vi "Indexed String To Enum.vi"(7 "Variant":variant, 8 "error in (no error)":errorcluster, 11 "String":string) -> (0 "error out":errorcluster, 3 "Enum":variant)   [LabVIEW 2017, in "ClusterCfgTable.lvlib"]
uses:
  ClusterCfgTable.lvlib
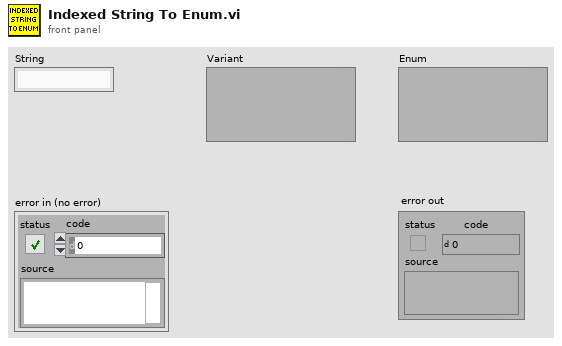
[diagram p1: front panel]
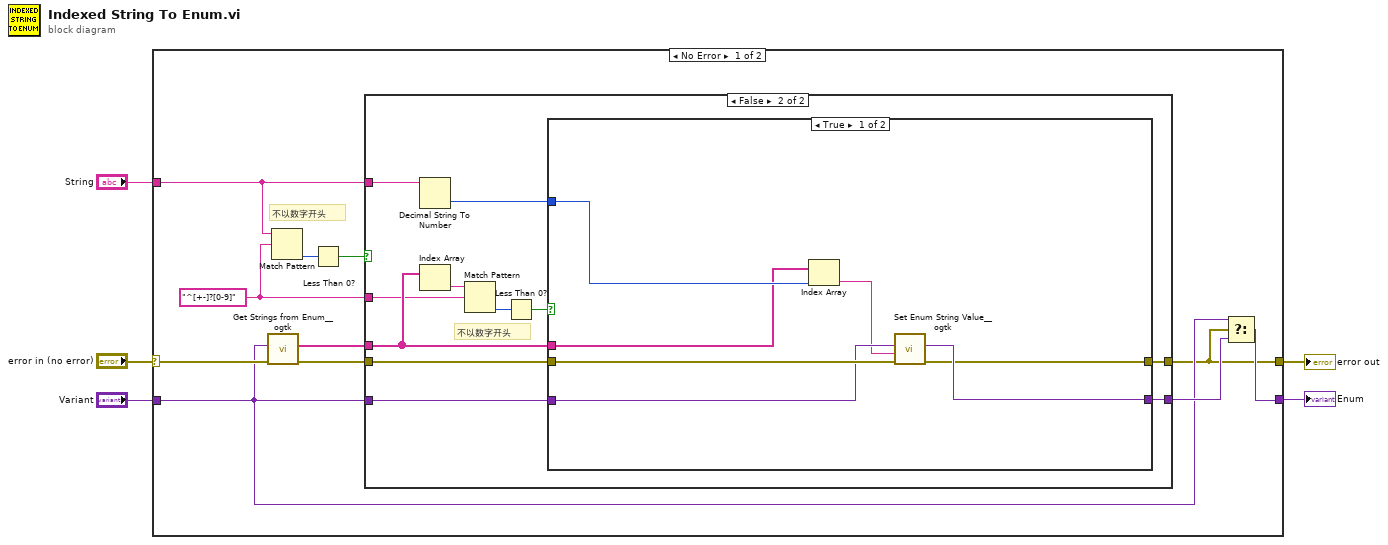
[diagram p0: block diagram]
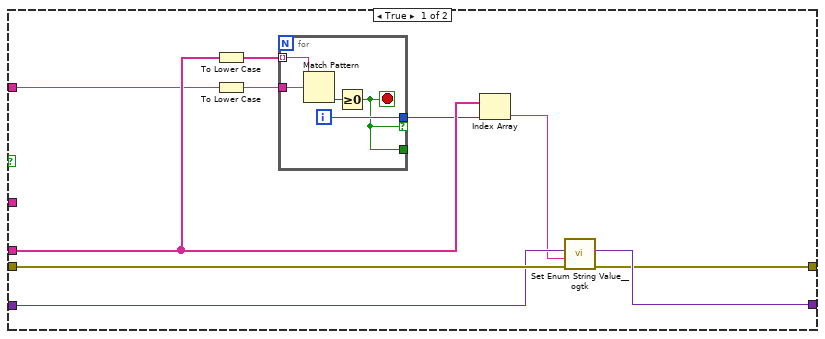
[diagram p2: hidden frame]
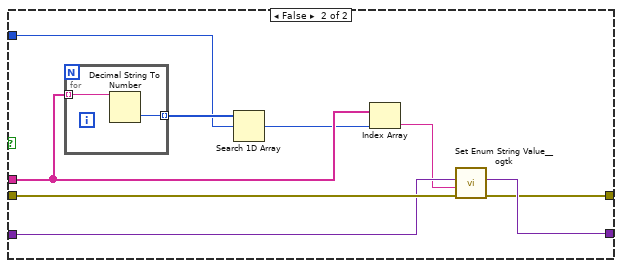
[diagram p3: hidden frame]
diagram:
  n1 = case shown="No Error" "error in (no error)" {
    selector: "error in (no error)" -> [w16 w62]
    tunnel: "Variant" -> [w8 w61]
    tunnel: "String" -> [w12 _]
    tunnel: [w7 w61] -> w2
    tunnel: [w6 w62] -> w1
    frame No Error {
      w10 = "^[+-]?[0-9]" ("regular expression")
      # "不以数字开头"
      n2 = call <userlib>:"Get Strings from Enum__ogtk.vi"("error in (no error)"=w16, "Enum"=w8) -> ("error out"=w15:errorcluster, "Enum Strings"=w14:string[])  [unwired: 6 in, 2 out]
      n3 = Match Pattern(string=w12, regular expression=w10) -> (offset past match=w13:i32)  [unwired: 1 in, 3 out]
      n4 = Less Than 0?(x=w13) -> (x < 0?=w11:bool)
      n5 = case shown="False" w11 {
        tunnel: [w26 w42] -> w9
        tunnel: w15 -> [w25 w41]
        tunnel: w8 -> [w24 w40]
        tunnel: [w23 w39] -> w6
        tunnel: w14 -> [w22 w37]
        tunnel: w12 -> [w19 w38]
        tunnel: w10 -> [_ w34]
        frame True {
          n6 = To Lower Case(string=w22) -> (all lower case string=w18:string[])
          n7 = To Lower Case(string=w19) -> (all lower case string=w17:string)
          n8 = for {
            tunnel: w18 -> [w31] mode=indexing
            tunnel: w17 -> [w30]
            tunnel: [w29] -> w21 if=w27
            tunnel: [w27] -> _
            i -> [w29]
            stop <- w27 stop-if-true
            n9 = Match Pattern(string=w31, regular expression=w30) -> (offset past match=w28:i32)  [unwired: 1 in, 3 out]
            n10 = Greater Or Equal To 0?(x=w28) -> (x >= 0?=w27:bool)
          }
          n11 = Index Array(array=w22, index=w21) -> (element=w20:string)
          n12 = call <userlib>:"Set Enum String Value__ogtk.vi"("error in (no error)"=w25, "String Value"=w20, "Default Enum Value"=w24) -> ("error out"=w23:errorcluster, "Enum"=w26:variant)  [unwired: 7 in]
        }
        frame False {
          # "不以数字开头"
          n13 = Decimal String To Number(string=w38) -> (number=w32:i32)  [unwired: 2 in, 1 out]
          n14 = Index Array(array=w37) -> (element=w35:string)  [unwired: 1 in]
          n15 = Match Pattern(string=w35, regular expression=w34) -> (offset past match=w36:i32)  [unwired: 1 in, 3 out]
          n16 = Less Than 0?(x=w36) -> (x < 0?=w33:bool)
          n17 = case shown="True" w33 {
            tunnel: [w49 w58] -> w42
            tunnel: w41 -> [w48 w57]
            tunnel: w40 -> [w47 w56]
            tunnel: [w46 w55] -> w39
            tunnel: w37 -> [w44 w54]
            tunnel: w32 -> [w45 w51]
            frame True {
              n18 = Index Array(array=w44, index=w45) -> (element=w43:string)
              n19 = call <userlib>:"Set Enum String Value__ogtk.vi"("error in (no error)"=w48, "String Value"=w43, "Default Enum Value"=w47) -> ("error out"=w46:errorcluster, "Enum"=w49:variant)  [unwired: 7 in]
            }
            frame False {
              n20 = for {
                tunnel: w54 -> [w60] mode=indexing
                tunnel: [w59] -> w52 mode=indexing
                n21 = Decimal String To Number(string=w60) -> (number=w59:i32)  [unwired: 2 in, 1 out]
              }
              n22 = Search 1D Array(1D array=w52, element=w51) -> (index of element=w50:i32)  [unwired: 1 in]
              n23 = Index Array(array=w54, index=w50) -> (element=w53:string)
              n24 = call <userlib>:"Set Enum String Value__ogtk.vi"("error in (no error)"=w57, "String Value"=w53, "Default Enum Value"=w56) -> ("error out"=w55:errorcluster, "Enum"=w58:variant)  [unwired: 7 in]
            }
          }
        }
      }
      n25 = Select(t=w8, s=w6, f=w9) -> (s? t:f=w7:variant)
    }
    frame Error {
    }
  }
  "Enum" <- w2
  "error out" <- w1
